vi "SERIAL_DecodePacket.vi"(10 "Data":u8[](array[numeric]), 11 "Packet":string) -> (2 "Data":u8[](array[numeric]), 3 "Packet":string)   [LabVIEW 2015, in "navX Library v1 (deprecated).lvlib"]
uses:
  navX Library v1 (deprecated).lvlib
  COMMON/TypeDefs/Value TypeDefs/navX NAVX_CAPABILITY_FLAGS.ctl
  COMMON/TypeDefs/Value TypeDefs/navX Device Registers.ctl
  TypeDefs/SERIAL_Device_Registers.ctl
  COMMON/Util/DataConvert/LabVIEW-to-navX/EncodeUnsignedHundredths.vi
  COMMON/Util/DataConvert/navX-to-LabVIEW/DecodeSignedHundredths.vi
  COMMON/Util/DataConvert/LabVIEW-to-navX/EncodeSignedHundredths.vi
  COMMON/Util/DataConvert/navX-to-LabVIEW/DecodeUInt16.vi
  COMMON/Util/DataConvert/navX-to-LabVIEW/DecodeInt16.vi
  COMMON/Util/DataConvert/navX-to-LabVIEW/DecodeUInt8.vi
  COMMON/Util/DataConvert/LabVIEW-to-navX/EncodeUInt16.vi
  COMMON/Util/DataConvert/navX-to-LabVIEW/DecodeUnsignedHundredths.vi
  COMMON/Util/DataConvert/navX-to-LabVIEW/DecodeSignedThousandths.vi
  COMMON/Util/DataConvert/LabVIEW-to-navX/EncodeSignedThousandths.vi
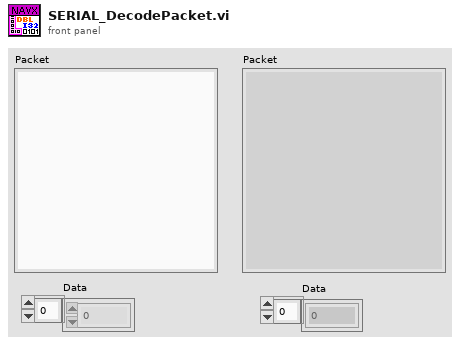
[diagram p1: front panel]
types:
  T1 = typedef "navX Library v1 (deprecated).lvlib/navX Device Registers.ctl" = u8
  T2 = typedef "navX Library v1 (deprecated).lvlib/navX NAVX_CAPABILITY_FLAGS.ctl" = u8
  T3 = typedef "navX Library v1 (deprecated).lvlib/SERIAL_Device_Registers.ctl" = u8
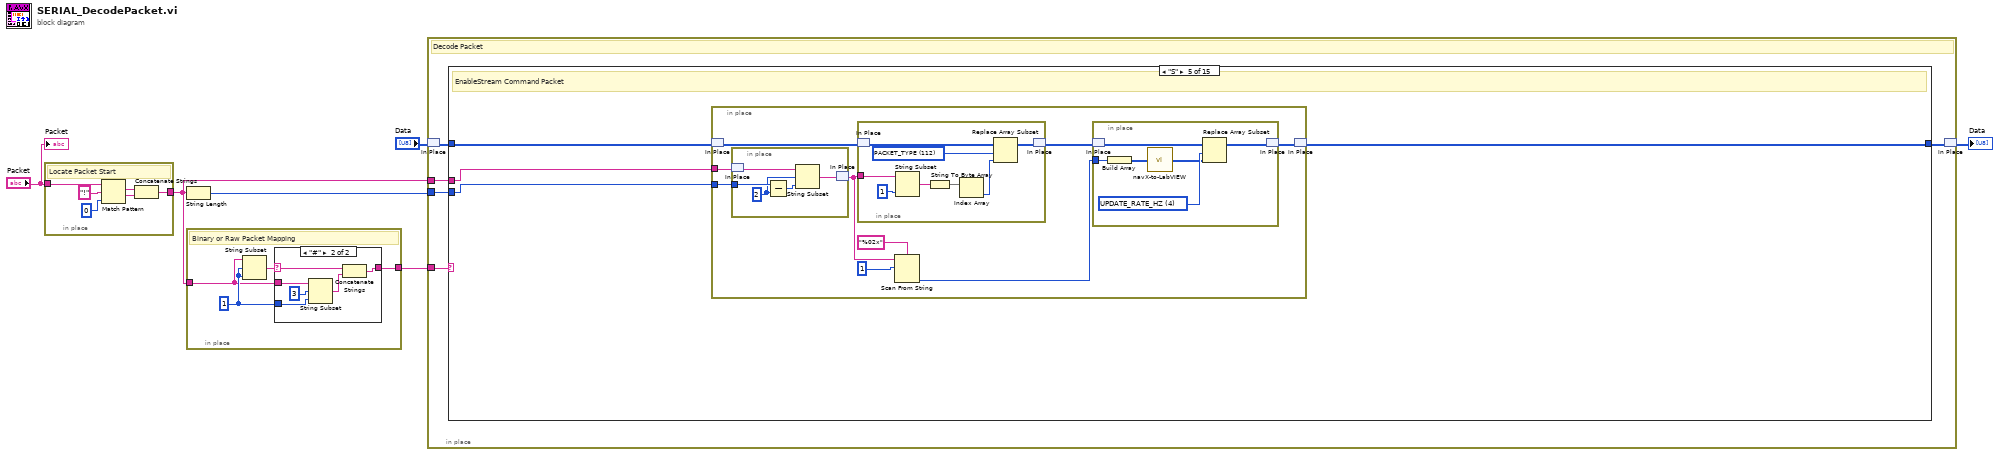
[diagram p0: block diagram]
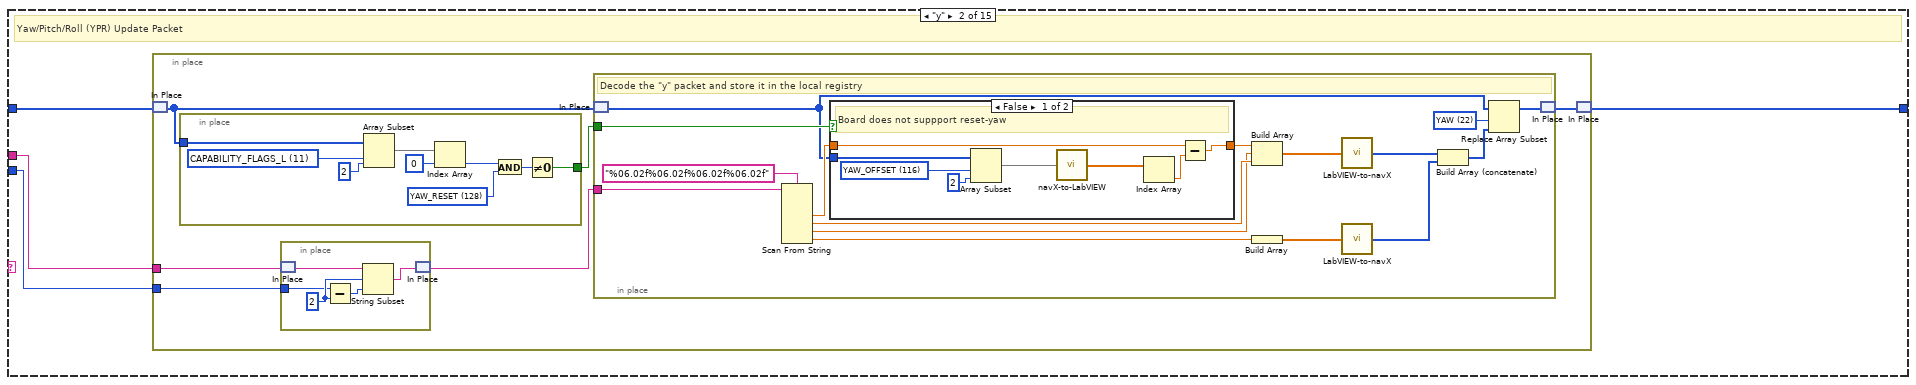
[diagram p3: hidden frame]
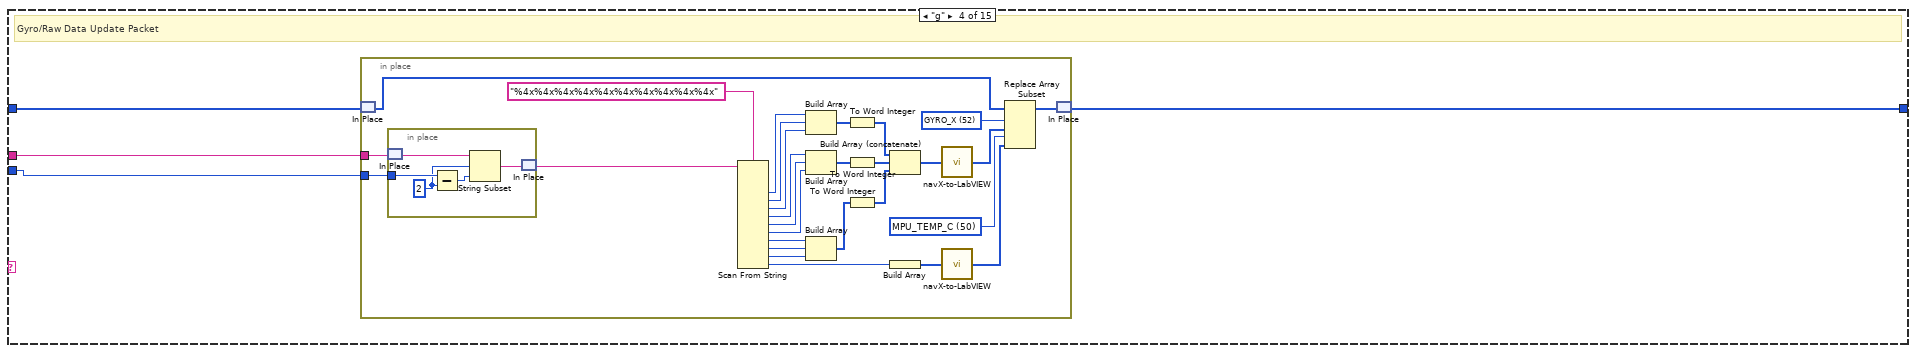
[diagram p6: hidden frame]
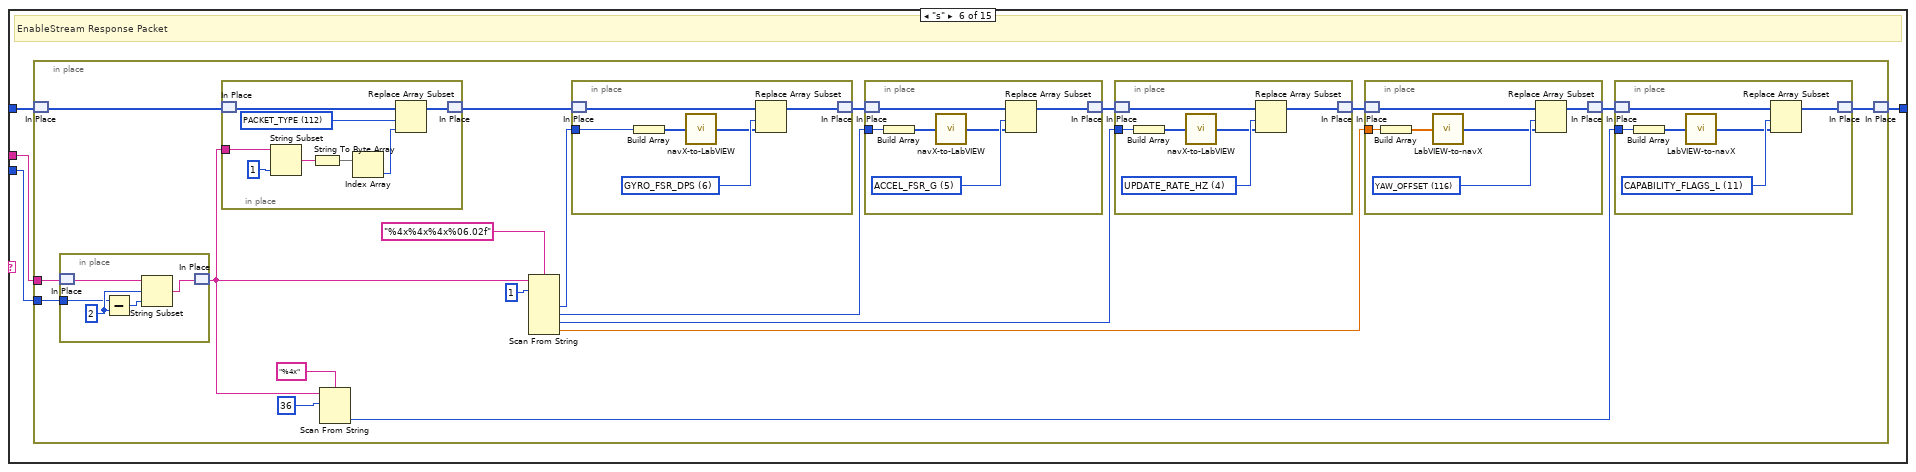
[diagram p7: hidden frame]
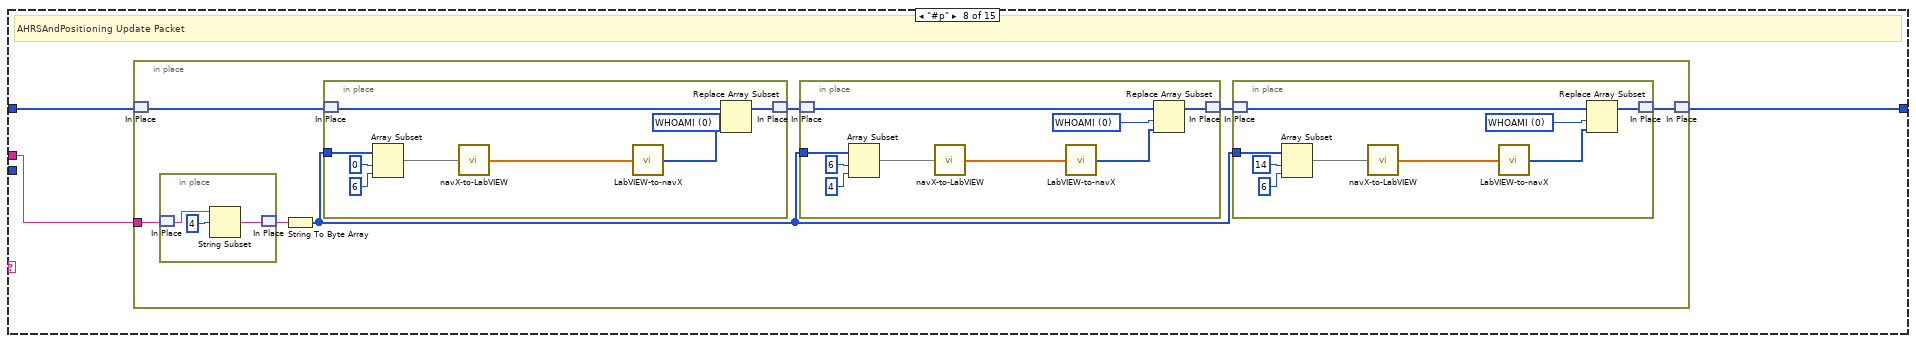
[diagram p9: hidden frame]
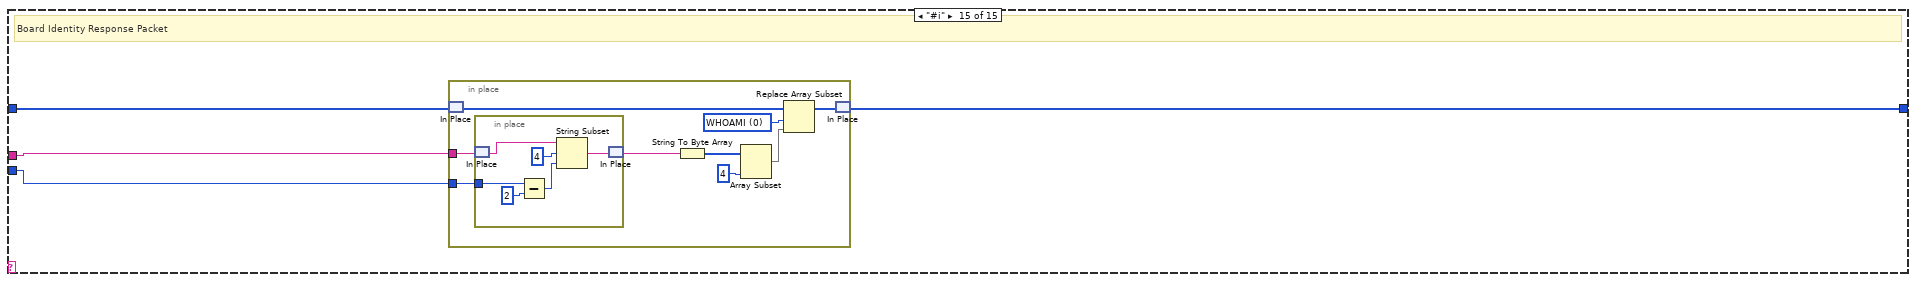
[diagram p16: hidden frame]
diagram:
  n1 = in-place {
    in-place-border: "Packet" -> [w11]
    in-place-border: [w8] -> w4
    # "Locate Packet Start"
    n2 = Match Pattern(string=w11, regular expression="!" ("Packet Start Char"), offset (0)=0 ("offset past match")) -> (match substring=w10:string, after substring=w9:string)  [unwired: 2 out]
    n3 = Concatenate Strings(w10, w9) -> (w8:string)
  }
  n4 = String Length(string=w4) -> (length=w3:i32)
  n5 = in-place {
    in-place-border: w4 -> [w14]
    in-place-border: [w16] -> w6
    w15 = 1 ("length (rest)")
    # "Binary or Raw Packet Mapping"
    n6 = String Subset(string=w14, offset (0)=w15, length (rest)=w15) -> (substring=w13:string)
    n7 = case shown="\"#\"" w13 {
      selector: w13 -> [w17 w18]
      tunnel: [w17 w19] -> w16
      tunnel: w15 -> [_ w22]
      tunnel: w14 -> [_ w21]
      frame Default {
      }
      frame "#" {
        n8 = String Subset(string=w21, offset (0)=3, length (rest)=w22) -> (substring=w20:string)
        n9 = Concatenate Strings(w18, w20) -> (w19:string)
      }
    }
  }
  n10 = in-place {
    in-place-border: w6 -> [w28]
    in-place-border: w4 -> [w27]
    in-place-border: w3 -> [w26]
    # "Decode Packet"
    n11 = in-place-match #1("Data") -> (w25:u8[])
    n12 = case shown="\"S\"" w28 {
      tunnel: w25 -> [w29 w31 w79 w81 w120 w150 w215 w217 w256 w257 w258 w259 w260 w261 w263]
      tunnel: [w29 w30 w79 w80 w119 w149 w215 w216 w256 w257 w258 w259 w260 w261 w262] -> w24
      tunnel: w27 -> [_ w32 _ w83 w118 w152 _ w218 _ _ _ _ _ _ w264]
      tunnel: w26 -> [_ w33 _ w82 w117 w151 _ _ _ _ _ _ _ _ w265]
      frame Default {
        # "Unknown Packet"
      }
      frame "y" {
        # "Yaw/Pitch/Roll (YPR) Update Packet"
        n13 = in-place {
          in-place-border: w33 -> [w38]
          in-place-border: w32 -> [w37]
          n14 = in-place-match #2(w31) -> (w35:u8[])
          n15 = in-place {
            in-place-border: w35 -> [w77]
            in-place-border: [w71] -> w39
            w70 = T1 11 items=["WHOAMI"=0, "HW_REV"=1, "FW_VER_MAJOR"=2, "FW_VER_MINOR"=3, "UPDATE_RATE_HZ"=4, "ACCEL_FSR_G"=5, "GYRO_FSR_DPS"=6, "OP_STATUS"=8, "CAL_STATUS"=9, "SELFTEST_STATUS"=10, "CAPABILITY_FLAGS_L"=11, "CAPABILITY_FLAGS_H"=12, "SENSOR_STATUS"=16, "TIMESTAMP"=18, "YAW"=22, "ROLL"=24, "PITCH"=26, "HEADING"=28, "FUSED_HEADING"=30, "ALTITUDE_I"=32, "ALTITUDE_D"=34, "LINERA_ACC_X"=36, "LINERA_ACC_Y"=38, "LINERA_ACC_Z"=40, "QUAT_W"=42, "QUAT_X"=44, "QUAT_Y"=46, "QUAT_Z"=48, "MPU_TEMP_C"=50, "GYRO_X"=52, "GYRO_Y"=54, "GYRO_Z"=56, "ACC_X"=58, "ACC_Y"=60, "ACC_Z"=62, "MAG_X"=64, "MAG_Y"=66, "MAG_Z"=68, "PRESSURE_I"=70, "PRESSURE_D"=72, "PRESSURE_TEMP"=74, "YAW_OFFSET"=76, "QUAT_OFFSET_W"=78, "QUAT_OFFSET_X"=80, "QUAT_OFFSET_Y"=82, "QUAT_OFFSET_Z"=84, "INTEGRATION_CONTROL"=86, "VELOCITY_X"=88, "VELOCITY_Y"=92, "VELOCITY_Z"=96, "DISPLACMENT_X"=100, "DISPLACMENT_Y"=104, "DISPLACEMENT_Z"=108] ("Device Register")
            w73 = T2 128 items=["OMNIMOUNT"=4, "VEL_AND_DISP "=64, "YAW_RESET"=128, "OMNIMOUNT_CONFIG_MASK"=56] ("NAVX_CAPABILITY_FLAG")
            n16 = Array Subset(array=w77, index=w70, length=2) -> (w75:u8[])
            n17 = Index Array(array=w75, index=u8 0 ("Read Size")) -> (element=w72:u8)
            n18 = And(x=w72, y=w73) -> (x .and. y?=w74:T2)
            n19 = Not Equal To 0?(x=w74) -> (x != 0?=w71:bool)
          }
          n20 = in-place {
            in-place-border: w38 -> [w67]
            w68 = 2 ("offset (0)")
            n21 = in-place-match #3(w37) -> (w65:string)
            n22 = Subtract(x=w67, y=w68) -> (x-y=w69:i32)
            n23 = String Subset(string=w65, offset (0)=w68, length (rest)=w69) -> (substring=w66:string)
            n24 = in-place-match #3(w66) -> (w36:string)
          }
          n25 = in-place {
            in-place-border: w39 -> [w53]
            in-place-border: w36 -> [w43]
            w44 = T1 22 items=["WHOAMI"=0, "HW_REV"=1, "FW_VER_MAJOR"=2, "FW_VER_MINOR"=3, "UPDATE_RATE_HZ"=4, "ACCEL_FSR_G"=5, "GYRO_FSR_DPS"=6, "OP_STATUS"=8, "CAL_STATUS"=9, "SELFTEST_STATUS"=10, "CAPABILITY_FLAGS_L"=11, "CAPABILITY_FLAGS_H"=12, "SENSOR_STATUS"=16, "TIMESTAMP"=18, "YAW"=22, "ROLL"=24, "PITCH"=26, "HEADING"=28, "FUSED_HEADING"=30, "ALTITUDE_I"=32, "ALTITUDE_D"=34, "LINERA_ACC_X"=36, "LINERA_ACC_Y"=38, "LINERA_ACC_Z"=40, "QUAT_W"=42, "QUAT_X"=44, "QUAT_Y"=46, "QUAT_Z"=48, "MPU_TEMP_C"=50, "GYRO_X"=52, "GYRO_Y"=54, "GYRO_Z"=56, "ACC_X"=58, "ACC_Y"=60, "ACC_Z"=62, "MAG_X"=64, "MAG_Y"=66, "MAG_Z"=68, "PRESSURE_I"=70, "PRESSURE_D"=72, "PRESSURE_TEMP"=74, "YAW_OFFSET"=76, "QUAT_OFFSET_W"=78, "QUAT_OFFSET_X"=80, "QUAT_OFFSET_Y"=82, "QUAT_OFFSET_Z"=84, "INTEGRATION_CONTROL"=86, "VELOCITY_X"=88, "VELOCITY_Y"=92, "VELOCITY_Z"=96, "DISPLACMENT_X"=100, "DISPLACMENT_Y"=104, "DISPLACEMENT_Z"=108] ("Device Register")
            # "Decode the \"y\" packet and store it in the local registry"
            n26 = in-place-match #4(w35) -> (w42:u8[])
            n27 = Scan From String(format string="%06.02f%06.02f%06.02f%06.02f", input string=w43) -> (output 1=w54:dbl, output 2=w46:dbl, output 3=w45:dbl, output 4=w48:dbl)  [unwired: 6 in, 3 out]
            n28 = case shown="False" w53 {
              tunnel: [w62 w64] -> w40
              tunnel: w54 -> [w63 w64]
              tunnel: w42 -> [w58 _]
              frame False {
                w60 = T3 116 items=["PACKET_TYPE"=112, "YAW_OFFSET"=116, "ROLL_OFFSET"=118, "PITCH_OFFSET"=120] ("Serial Device Register")
                # "Board does not suppport reset-yaw"
                n29 = Array Subset(array=w58, index=w60, length=2) -> (w59:u8[])
                n30 = call-poly "navX-to-LabVIEW.vi"("Data In"=w59) -> ("Data Out"=w57:dbl[])
                n31 = Index Array(array=w57) -> (element=w56:dbl)  [unwired: 1 in]
                n32 = Subtract(x=w63, y=w56) -> (x-y=w62:dbl)
              }
              frame True {
                # "Board does  suppport reset-yaw"
              }
            }
            n33 = Build Array(w40, w45, w46) -> (w52:dbl[])
            n34 = Build Array(w48) -> (w47:dbl[])
            n35 = call-poly "LabVIEW-to-navX.vi"("Data In"=w52) -> ("Data Out"=w51:u8[])
            n36 = call-poly "LabVIEW-to-navX.vi"("Data In"=w47) -> ("Data Out"=w50:u8[])
            n37 = Build Array (concatenate)(w51, w50) -> (w49:u8[])
            n38 = Replace Array Subset(array=w42, new element=w49, index=w44) -> (w41:u8[])
            n39 = in-place-match #4(w41) -> (w34:u8[])
          }
          n40 = in-place-match #2(w34) -> (w30:u8[])
        }
      }
      frame "q" {
        # "Quaternion Update Packet"
      }
      frame "g" {
        # "Gyro/Raw Data Update Packet"
        n41 = in-place {
          in-place-border: w83 -> [w85]
          in-place-border: w82 -> [w110]
          w88 = T1 50 items=["WHOAMI"=0, "HW_REV"=1, "FW_VER_MAJOR"=2, "FW_VER_MINOR"=3, "UPDATE_RATE_HZ"=4, "ACCEL_FSR_G"=5, "GYRO_FSR_DPS"=6, "OP_STATUS"=8, "CAL_STATUS"=9, "SELFTEST_STATUS"=10, "CAPABILITY_FLAGS_L"=11, "CAPABILITY_FLAGS_H"=12, "SENSOR_STATUS"=16, "TIMESTAMP"=18, "YAW"=22, "PITCH"=24, "ROLL"=26, "HEADING"=28, "FUSED_HEADING"=30, "ALTITUDE_I"=32, "ALTITUDE_D"=34, "LINERA_ACC_X"=36, "LINERA_ACC_Y"=38, "LINERA_ACC_Z"=40, "QUAT_W"=42, "QUAT_X"=44, "QUAT_Y"=46, "QUAT_Z"=48, "MPU_TEMP_C"=50, "GYRO_X"=52, "GYRO_Y"=54, "GYRO_Z"=56, "ACC_X"=58, "ACC_Y"=60, "ACC_Z"=62, "MAG_X"=64, "MAG_Y"=66, "MAG_Z"=68, "PRESSURE_I"=70, "PRESSURE_D"=72, "PRESSURE_TEMP"=74, "YAW_OFFSET"=76, "QUAT_OFFSET_W"=78, "QUAT_OFFSET_X"=80, "QUAT_OFFSET_Y"=82, "QUAT_OFFSET_Z"=84, "INTEGRATION_CONTROL"=86, "VELOCITY_X"=88, "VELOCITY_Y"=92, "VELOCITY_Z"=96, "DISPLACMENT_X"=100, "DISPLACMENT_Y"=104, "DISPLACEMENT_Z"=108] ("Device Register")
          w111 = T1 52 items=["WHOAMI"=0, "HW_REV"=1, "FW_VER_MAJOR"=2, "FW_VER_MINOR"=3, "UPDATE_RATE_HZ"=4, "ACCEL_FSR_G"=5, "GYRO_FSR_DPS"=6, "OP_STATUS"=8, "CAL_STATUS"=9, "SELFTEST_STATUS"=10, "CAPABILITY_FLAGS_L"=11, "CAPABILITY_FLAGS_H"=12, "SENSOR_STATUS"=16, "TIMESTAMP"=18, "YAW"=22, "PITCH"=24, "ROLL"=26, "HEADING"=28, "FUSED_HEADING"=30, "ALTITUDE_I"=32, "ALTITUDE_D"=34, "LINERA_ACC_X"=36, "LINERA_ACC_Y"=38, "LINERA_ACC_Z"=40, "QUAT_W"=42, "QUAT_X"=44, "QUAT_Y"=46, "QUAT_Z"=48, "MPU_TEMP_C"=50, "GYRO_X"=52, "GYRO_Y"=54, "GYRO_Z"=56, "ACC_X"=58, "ACC_Y"=60, "ACC_Z"=62, "MAG_X"=64, "MAG_Y"=66, "MAG_Z"=68, "PRESSURE_I"=70, "PRESSURE_D"=72, "PRESSURE_TEMP"=74, "YAW_OFFSET"=76, "QUAT_OFFSET_W"=78, "QUAT_OFFSET_X"=80, "QUAT_OFFSET_Y"=82, "QUAT_OFFSET_Z"=84, "INTEGRATION_CONTROL"=86, "VELOCITY_X"=88, "VELOCITY_Y"=92, "VELOCITY_Z"=96, "DISPLACMENT_X"=100, "DISPLACMENT_Y"=104, "DISPLACEMENT_Z"=108] ("Device Register")
          n42 = in-place-match #5(w81) -> (w93:u8[])
          n43 = in-place {
            in-place-border: w110 -> [w116]
            w114 = 2 ("offset (0)")
            n44 = in-place-match #6(w85) -> (w113:string)
            n45 = Subtract(x=w116, y=w114) -> (x-y=w115:i32)
            n46 = String Subset(string=w113, offset (0)=w114, length (rest)=w115) -> (substring=w112:string)
            n47 = in-place-match #6(w112) -> (w84:string)
          }
          n48 = Scan From String(format string="%4x%4x%4x%4x%4x%4x%4x%4x%4x%4x", input string=w84) -> (output 1=w108:u32, output 2=w107:u32, output 3=w106:u32, output 4=w105:u32, output 5=w104:u32, output 6=w103:u32, output 7=w102:u32, output 8=w101:u32, output 9=w100:u32, output 10=w91:u32)  [unwired: 12 in, 3 out]
          n49 = Build Array(w108, w107, w106) -> (w97:u32[])
          n50 = Build Array(w105, w104, w103) -> (w99:u32[])
          n51 = Build Array(w102, w101, w100) -> (w98:u32[])
          n52 = To Word Integer(number=w97) -> (16bit integer=w96:i16[])
          n53 = To Word Integer(number=w99) -> (16bit integer=w95:i16[])
          n54 = To Word Integer(number=w98) -> (16bit integer=w92:i16[])
          n55 = Build Array (concatenate)(w96, w95, w92) -> (w87:i16[])
          n56 = Build Array(w91) -> (w90:u32[])
          n57 = call-poly "navX-to-LabVIEW.vi"("Data In"=w87) -> ("Data Out"=w86:i16[])
          n58 = call-poly "navX-to-LabVIEW.vi"("Data In"=w90) -> ("Data Out"=w89:u16[])
          n59 = Replace Array Subset(array=w93, new element #1=w86, index #1=w111, new element #2=w89, index #2=w88) -> (w94:u8[])
          n60 = in-place-match #5(w94) -> (w80:u8[])
        }
      }
      frame "S" {
        # "EnableStream Command Packet"
        n61 = in-place {
          in-place-border: w118 -> [w128]
          in-place-border: w117 -> [w127]
          n62 = in-place-match #7(w120) -> (w129:u8[])
          n63 = in-place {
            in-place-border: w127 -> [w140]
            w138 = 2 ("offset (0)")
            n64 = in-place-match #8(w128) -> (w137:string)
            n65 = Subtract(x=w140, y=w138) -> (x-y=w139:i32)
            n66 = String Subset(string=w137, offset (0)=w138, length (rest)=w139) -> (substring=w136:string)
            n67 = in-place-match #8(w136) -> (w126:string)
          }
          n68 = in-place {
            in-place-border: w126 -> [w148]
            w143 = T3 112 items=["PACKET_TYPE"=112, "YAW_OFFSET"=116, "ROLL_OFFSET"=118, "PITCH_OFFSET"=120] ("Serial Device Register")
            n69 = in-place-match #9(w129) -> (w144:u8[])
            n70 = String Subset(string=w148, length (rest)=1 ("length (rest)")) -> (substring=w146:string)  [unwired: 1 in]
            n71 = String To Byte Array(string=w146) -> (unsigned byte array=w145:u8[])
            n72 = Index Array(array=w145) -> (element=w142:u8)  [unwired: 1 in]
            n73 = Replace Array Subset(array=w144, new element=w142, index=w143) -> (w141:u8[])
            n74 = in-place-match #9(w141) -> (w121:u8[])
          }
          n75 = Scan From String(format string="%02x", input string=w126, initial scan location=u32 1) -> (output 1=w123:u32)  [unwired: 2 in, 3 out]
          n76 = in-place {
            in-place-border: w123 -> [w135]
            w133 = T1 4 items=["WHOAMI"=0, "HW_REV"=1, "FW_VER_MAJOR"=2, "FW_VER_MINOR"=3, "UPDATE_RATE_HZ"=4, "ACCEL_FSR_G"=5, "GYRO_FSR_DPS"=6, "OP_STATUS"=8, "CAL_STATUS"=9, "SELFTEST_STATUS"=10, "CAPABILITY_FLAGS_L"=11, "CAPABILITY_FLAGS_H"=12, "SENSOR_STATUS"=16, "TIMESTAMP"=18, "YAW"=22, "PITCH"=24, "ROLL"=26, "HEADING"=28, "FUSED_HEADING"=30, "ALTITUDE_I"=32, "ALTITUDE_D"=34, "LINERA_ACC_X"=36, "LINERA_ACC_Y"=38, "LINERA_ACC_Z"=40, "QUAT_W"=42, "QUAT_X"=44, "QUAT_Y"=46, "QUAT_Z"=48, "MPU_TEMP_C"=50, "GYRO_X"=52, "GYRO_Y"=54, "GYRO_Z"=56, "ACC_X"=58, "ACC_Y"=60, "ACC_Z"=62, "MAG_X"=64, "MAG_Y"=66, "MAG_Z"=68, "PRESSURE_I"=70, "PRESSURE_D"=72, "PRESSURE_TEMP"=74, "YAW_OFFSET"=76, "QUAT_OFFSET_W"=78, "QUAT_OFFSET_X"=80, "QUAT_OFFSET_Y"=82, "QUAT_OFFSET_Z"=84, "INTEGRATION_CONTROL"=86, "VELOCITY_X"=88, "VELOCITY_Y"=92, "VELOCITY_Z"=96, "DISPLACMENT_X"=100, "DISPLACMENT_Y"=104, "DISPLACEMENT_Z"=108] ("Device Register")
            n77 = in-place-match #10(w121) -> (w131:u8[])
            n78 = Build Array(w135) -> (w134:u32[])
            n79 = call-poly "navX-to-LabVIEW.vi"("Data In"=w134) -> ("Data Out"=w132:u8[])
            n80 = Replace Array Subset(array=w131, new element=w132, index=w133) -> (w130:u8[])
            n81 = in-place-match #10(w130) -> (w122:u8[])
          }
          n82 = in-place-match #7(w122) -> (w119:u8[])
        }
      }
      frame "s" {
        # "EnableStream Response Packet"
        n83 = in-place {
          in-place-border: w152 -> [w166]
          in-place-border: w151 -> [w170]
          n84 = in-place-match #11(w150) -> (w165:u8[])
          n85 = in-place {
            in-place-border: w170 -> [w212]
            w213 = 2 ("offset (0)")
            n86 = in-place-match #12(w166) -> (w211:string)
            n87 = Subtract(x=w212, y=w213) -> (x-y=w214:i32)
            n88 = String Subset(string=w211, offset (0)=w213, length (rest)=w214) -> (substring=w210:string)
            n89 = in-place-match #12(w210) -> (w164:string)
          }
          n90 = in-place {
            in-place-border: w164 -> [w209]
            w204 = T3 112 items=["PACKET_TYPE"=112, "YAW_OFFSET"=116, "ROLL_OFFSET"=118, "PITCH_OFFSET"=120] ("Serial Device Register")
            n91 = in-place-match #13(w165) -> (w205:u8[])
            n92 = String Subset(string=w209, length (rest)=1 ("length (rest)")) -> (substring=w207:string)  [unwired: 1 in]
            n93 = String To Byte Array(string=w207) -> (unsigned byte array=w206:u8[])
            n94 = Index Array(array=w206) -> (element=w203:u8)  [unwired: 1 in]
            n95 = Replace Array Subset(array=w205, new element=w203, index=w204) -> (w202:u8[])
            n96 = in-place-match #13(w202) -> (w163:u8[])
          }
          n97 = Scan From String(format string="%4x", input string=w164, initial scan location=u32 36) -> (output 1=w154:u32)  [unwired: 2 in, 3 out]
          n98 = Scan From String(format string="%4x%4x%4x%06.02f", input string=w164, initial scan location=u32 1) -> (output 1=w161:u32, output 2=w160:u32, output 3=w158:u32, output 4=w156:dbl)  [unwired: 5 in, 3 out]
          n99 = in-place {
            in-place-border: w161 -> [w201]
            w199 = T1 6 items=["WHOAMI"=0, "HW_REV"=1, "FW_VER_MAJOR"=2, "FW_VER_MINOR"=3, "UPDATE_RATE_HZ"=4, "ACCEL_FSR_G"=5, "GYRO_FSR_DPS"=6, "OP_STATUS"=8, "CAL_STATUS"=9, "SELFTEST_STATUS"=10, "CAPABILITY_FLAGS_L"=11, "CAPABILITY_FLAGS_H"=12, "SENSOR_STATUS"=16, "TIMESTAMP"=18, "YAW"=22, "PITCH"=24, "ROLL"=26, "HEADING"=28, "FUSED_HEADING"=30, "ALTITUDE_I"=32, "ALTITUDE_D"=34, "LINERA_ACC_X"=36, "LINERA_ACC_Y"=38, "LINERA_ACC_Z"=40, "QUAT_W"=42, "QUAT_X"=44, "QUAT_Y"=46, "QUAT_Z"=48, "MPU_TEMP_C"=50, "GYRO_X"=52, "GYRO_Y"=54, "GYRO_Z"=56, "ACC_X"=58, "ACC_Y"=60, "ACC_Z"=62, "MAG_X"=64, "MAG_Y"=66, "MAG_Z"=68, "PRESSURE_I"=70, "PRESSURE_D"=72, "PRESSURE_TEMP"=74, "YAW_OFFSET"=76, "QUAT_OFFSET_W"=78, "QUAT_OFFSET_X"=80, "QUAT_OFFSET_Y"=82, "QUAT_OFFSET_Z"=84, "INTEGRATION_CONTROL"=86, "VELOCITY_X"=88, "VELOCITY_Y"=92, "VELOCITY_Z"=96, "DISPLACMENT_X"=100, "DISPLACMENT_Y"=104, "DISPLACEMENT_Z"=108] ("Device Register")
            n100 = in-place-match #14(w163) -> (w197:u8[])
            n101 = Build Array(w201) -> (w200:u32[])
            n102 = call-poly "navX-to-LabVIEW.vi"("Data In"=w200) -> ("Data Out"=w198:u16[])
            n103 = Replace Array Subset(array=w197, new element=w198, index=w199) -> (w196:u8[])
            n104 = in-place-match #14(w196) -> (w162:u8[])
          }
          n105 = in-place {
            in-place-border: w160 -> [w195]
            w193 = T1 5 items=["WHOAMI"=0, "HW_REV"=1, "FW_VER_MAJOR"=2, "FW_VER_MINOR"=3, "UPDATE_RATE_HZ"=4, "ACCEL_FSR_G"=5, "GYRO_FSR_DPS"=6, "OP_STATUS"=8, "CAL_STATUS"=9, "SELFTEST_STATUS"=10, "CAPABILITY_FLAGS_L"=11, "CAPABILITY_FLAGS_H"=12, "SENSOR_STATUS"=16, "TIMESTAMP"=18, "YAW"=22, "PITCH"=24, "ROLL"=26, "HEADING"=28, "FUSED_HEADING"=30, "ALTITUDE_I"=32, "ALTITUDE_D"=34, "LINERA_ACC_X"=36, "LINERA_ACC_Y"=38, "LINERA_ACC_Z"=40, "QUAT_W"=42, "QUAT_X"=44, "QUAT_Y"=46, "QUAT_Z"=48, "MPU_TEMP_C"=50, "GYRO_X"=52, "GYRO_Y"=54, "GYRO_Z"=56, "ACC_X"=58, "ACC_Y"=60, "ACC_Z"=62, "MAG_X"=64, "MAG_Y"=66, "MAG_Z"=68, "PRESSURE_I"=70, "PRESSURE_D"=72, "PRESSURE_TEMP"=74, "YAW_OFFSET"=76, "QUAT_OFFSET_W"=78, "QUAT_OFFSET_X"=80, "QUAT_OFFSET_Y"=82, "QUAT_OFFSET_Z"=84, "INTEGRATION_CONTROL"=86, "VELOCITY_X"=88, "VELOCITY_Y"=92, "VELOCITY_Z"=96, "DISPLACMENT_X"=100, "DISPLACMENT_Y"=104, "DISPLACEMENT_Z"=108] ("Device Register")
            n106 = in-place-match #15(w162) -> (w191:u8[])
            n107 = Build Array(w195) -> (w194:u32[])
            n108 = call-poly "navX-to-LabVIEW.vi"("Data In"=w194) -> ("Data Out"=w192:u16[])
            n109 = Replace Array Subset(array=w191, new element=w192, index=w193) -> (w190:u8[])
            n110 = in-place-match #15(w190) -> (w159:u8[])
          }
          n111 = in-place {
            in-place-border: w158 -> [w189]
            w187 = T1 4 items=["WHOAMI"=0, "HW_REV"=1, "FW_VER_MAJOR"=2, "FW_VER_MINOR"=3, "UPDATE_RATE_HZ"=4, "ACCEL_FSR_G"=5, "GYRO_FSR_DPS"=6, "OP_STATUS"=8, "CAL_STATUS"=9, "SELFTEST_STATUS"=10, "CAPABILITY_FLAGS_L"=11, "CAPABILITY_FLAGS_H"=12, "SENSOR_STATUS"=16, "TIMESTAMP"=18, "YAW"=22, "PITCH"=24, "ROLL"=26, "HEADING"=28, "FUSED_HEADING"=30, "ALTITUDE_I"=32, "ALTITUDE_D"=34, "LINERA_ACC_X"=36, "LINERA_ACC_Y"=38, "LINERA_ACC_Z"=40, "QUAT_W"=42, "QUAT_X"=44, "QUAT_Y"=46, "QUAT_Z"=48, "MPU_TEMP_C"=50, "GYRO_X"=52, "GYRO_Y"=54, "GYRO_Z"=56, "ACC_X"=58, "ACC_Y"=60, "ACC_Z"=62, "MAG_X"=64, "MAG_Y"=66, "MAG_Z"=68, "PRESSURE_I"=70, "PRESSURE_D"=72, "PRESSURE_TEMP"=74, "YAW_OFFSET"=76, "QUAT_OFFSET_W"=78, "QUAT_OFFSET_X"=80, "QUAT_OFFSET_Y"=82, "QUAT_OFFSET_Z"=84, "INTEGRATION_CONTROL"=86, "VELOCITY_X"=88, "VELOCITY_Y"=92, "VELOCITY_Z"=96, "DISPLACMENT_X"=100, "DISPLACMENT_Y"=104, "DISPLACEMENT_Z"=108] ("Device Register")
            n112 = in-place-match #16(w159) -> (w185:u8[])
            n113 = Build Array(w189) -> (w188:u32[])
            n114 = call-poly "navX-to-LabVIEW.vi"("Data In"=w188) -> ("Data Out"=w186:u8[])
            n115 = Replace Array Subset(array=w185, new element=w186, index=w187) -> (w184:u8[])
            n116 = in-place-match #16(w184) -> (w157:u8[])
          }
          n117 = in-place {
            in-place-border: w156 -> [w183]
            w181 = T3 116 items=["PACKET_TYPE"=112, "YAW_OFFSET"=116, "ROLL_OFFSET"=118, "PITCH_OFFSET"=120] ("Serial Device Register")
            n118 = in-place-match #17(w157) -> (w179:u8[])
            n119 = Build Array(w183) -> (w182:dbl[])
            n120 = call-poly "LabVIEW-to-navX.vi"("Data In"=w182) -> ("Data Out"=w180:u8[])
            n121 = Replace Array Subset(array=w179, new element=w180, index=w181) -> (w178:u8[])
            n122 = in-place-match #17(w178) -> (w155:u8[])
          }
          n123 = in-place {
            in-place-border: w154 -> [w177]
            w175 = T1 11 items=["WHOAMI"=0, "HW_REV"=1, "FW_VER_MAJOR"=2, "FW_VER_MINOR"=3, "UPDATE_RATE_HZ"=4, "ACCEL_FSR_G"=5, "GYRO_FSR_DPS"=6, "OP_STATUS"=8, "CAL_STATUS"=9, "SELFTEST_STATUS"=10, "CAPABILITY_FLAGS_L"=11, "CAPABILITY_FLAGS_H"=12, "SENSOR_STATUS"=16, "TIMESTAMP"=18, "YAW"=22, "PITCH"=24, "ROLL"=26, "HEADING"=28, "FUSED_HEADING"=30, "ALTITUDE_I"=32, "ALTITUDE_D"=34, "LINERA_ACC_X"=36, "LINERA_ACC_Y"=38, "LINERA_ACC_Z"=40, "QUAT_W"=42, "QUAT_X"=44, "QUAT_Y"=46, "QUAT_Z"=48, "MPU_TEMP_C"=50, "GYRO_X"=52, "GYRO_Y"=54, "GYRO_Z"=56, "ACC_X"=58, "ACC_Y"=60, "ACC_Z"=62, "MAG_X"=64, "MAG_Y"=66, "MAG_Z"=68, "PRESSURE_I"=70, "PRESSURE_D"=72, "PRESSURE_TEMP"=74, "YAW_OFFSET"=76, "QUAT_OFFSET_W"=78, "QUAT_OFFSET_X"=80, "QUAT_OFFSET_Y"=82, "QUAT_OFFSET_Z"=84, "INTEGRATION_CONTROL"=86, "VELOCITY_X"=88, "VELOCITY_Y"=92, "VELOCITY_Z"=96, "DISPLACMENT_X"=100, "DISPLACMENT_Y"=104, "DISPLACEMENT_Z"=108] ("Device Register")
            n124 = in-place-match #18(w155) -> (w173:u8[])
            n125 = Build Array(w177) -> (w176:u32[])
            n126 = call-poly "LabVIEW-to-navX.vi"("Data In"=w176) -> ("Data Out"=w174:u8[])
            n127 = Replace Array Subset(array=w173, new element=w174, index=w175) -> (w172:u8[])
            n128 = in-place-match #18(w172) -> (w153:u8[])
          }
          n129 = in-place-match #11(w153) -> (w149:u8[])
        }
      }
      frame "#a" {
        # "AHRS Update Packet"
      }
      frame "#p" {
        # "AHRSAndPositioning Update Packet"
        n130 = in-place {
          in-place-border: w218 -> [w222]
          n131 = in-place-match #19(w217) -> (w220:u8[])
          n132 = in-place {
            n133 = in-place-match #20(w222) -> (w228:string)
            n134 = String Subset(string=w228, offset (0)=4) -> (substring=w226:string)  [unwired: 1 in]
            n135 = in-place-match #20(w226) -> (w221:string)
          }
          n136 = String To Byte Array(string=w221) -> (unsigned byte array=w223:u8[])
          n137 = in-place {
            in-place-border: w223 -> [w252]
            w247 = T1 0 items=["WHOAMI"=0, "HW_REV"=1, "FW_VER_MAJOR"=2, "FW_VER_MINOR"=3, "UPDATE_RATE_HZ"=4, "ACCEL_FSR_G"=5, "GYRO_FSR_DPS"=6, "OP_STATUS"=8, "CAL_STATUS"=9, "SELFTEST_STATUS"=10, "CAPABILITY_FLAGS_L"=11, "CAPABILITY_FLAGS_H"=12, "SENSOR_STATUS"=16, "TIMESTAMP"=18, "YAW"=22, "PITCH"=24, "ROLL"=26, "HEADING"=28, "FUSED_HEADING"=30, "ALTITUDE_I"=32, "ALTITUDE_D"=34, "LINERA_ACC_X"=36, "LINERA_ACC_Y"=38, "LINERA_ACC_Z"=40, "QUAT_W"=42, "QUAT_X"=44, "QUAT_Y"=46, "QUAT_Z"=48, "MPU_TEMP_C"=50, "GYRO_X"=52, "GYRO_Y"=54, "GYRO_Z"=56, "ACC_X"=58, "ACC_Y"=60, "ACC_Z"=62, "MAG_X"=64, "MAG_Y"=66, "MAG_Z"=68, "PRESSURE_I"=70, "PRESSURE_D"=72, "PRESSURE_TEMP"=74, "YAW_OFFSET"=76, "QUAT_OFFSET_W"=78, "QUAT_OFFSET_X"=80, "QUAT_OFFSET_Y"=82, "QUAT_OFFSET_Z"=84, "INTEGRATION_CONTROL"=86, "VELOCITY_X"=88, "VELOCITY_Y"=92, "VELOCITY_Z"=96, "DISPLACMENT_X"=100, "DISPLACMENT_Y"=104, "DISPLACEMENT_Z"=108] ("Device Register")
            n138 = in-place-match #21(w220) -> (w250:u8[])
            n139 = Array Subset(array=w252, index=0, length=6) -> (w255:u8[])
            n140 = call-poly "navX-to-LabVIEW.vi"("Data In"=w255) -> ("Data Out"=w251:dbl[])
            n141 = call-poly "LabVIEW-to-navX.vi"("Data In"=w251) -> ("Data Out"=w249:u8[])
            n142 = Replace Array Subset(array=w250, new element=w249, index=w247) -> (w248:u8[])
            n143 = in-place-match #21(w248) -> (w225:u8[])
          }
          n144 = in-place {
            in-place-border: w223 -> [w243]
            w238 = T1 0 items=["WHOAMI"=0, "HW_REV"=1, "FW_VER_MAJOR"=2, "FW_VER_MINOR"=3, "UPDATE_RATE_HZ"=4, "ACCEL_FSR_G"=5, "GYRO_FSR_DPS"=6, "OP_STATUS"=8, "CAL_STATUS"=9, "SELFTEST_STATUS"=10, "CAPABILITY_FLAGS_L"=11, "CAPABILITY_FLAGS_H"=12, "SENSOR_STATUS"=16, "TIMESTAMP"=18, "YAW"=22, "PITCH"=24, "ROLL"=26, "HEADING"=28, "FUSED_HEADING"=30, "ALTITUDE_I"=32, "ALTITUDE_D"=34, "LINERA_ACC_X"=36, "LINERA_ACC_Y"=38, "LINERA_ACC_Z"=40, "QUAT_W"=42, "QUAT_X"=44, "QUAT_Y"=46, "QUAT_Z"=48, "MPU_TEMP_C"=50, "GYRO_X"=52, "GYRO_Y"=54, "GYRO_Z"=56, "ACC_X"=58, "ACC_Y"=60, "ACC_Z"=62, "MAG_X"=64, "MAG_Y"=66, "MAG_Z"=68, "PRESSURE_I"=70, "PRESSURE_D"=72, "PRESSURE_TEMP"=74, "YAW_OFFSET"=76, "QUAT_OFFSET_W"=78, "QUAT_OFFSET_X"=80, "QUAT_OFFSET_Y"=82, "QUAT_OFFSET_Z"=84, "INTEGRATION_CONTROL"=86, "VELOCITY_X"=88, "VELOCITY_Y"=92, "VELOCITY_Z"=96, "DISPLACMENT_X"=100, "DISPLACMENT_Y"=104, "DISPLACEMENT_Z"=108] ("Device Register")
            n145 = in-place-match #22(w225) -> (w241:u8[])
            n146 = Array Subset(array=w243, index=6, length=4) -> (w246:u8[])
            n147 = call-poly "navX-to-LabVIEW.vi"("Data In"=w246) -> ("Data Out"=w242:dbl[])
            n148 = call-poly "LabVIEW-to-navX.vi"("Data In"=w242) -> ("Data Out"=w240:u8[])
            n149 = Replace Array Subset(array=w241, new element=w240, index=w238) -> (w239:u8[])
            n150 = in-place-match #22(w239) -> (w224:u8[])
          }
          n151 = in-place {
            in-place-border: w223 -> [w234]
            w229 = T1 0 items=["WHOAMI"=0, "HW_REV"=1, "FW_VER_MAJOR"=2, "FW_VER_MINOR"=3, "UPDATE_RATE_HZ"=4, "ACCEL_FSR_G"=5, "GYRO_FSR_DPS"=6, "OP_STATUS"=8, "CAL_STATUS"=9, "SELFTEST_STATUS"=10, "CAPABILITY_FLAGS_L"=11, "CAPABILITY_FLAGS_H"=12, "SENSOR_STATUS"=16, "TIMESTAMP"=18, "YAW"=22, "PITCH"=24, "ROLL"=26, "HEADING"=28, "FUSED_HEADING"=30, "ALTITUDE_I"=32, "ALTITUDE_D"=34, "LINERA_ACC_X"=36, "LINERA_ACC_Y"=38, "LINERA_ACC_Z"=40, "QUAT_W"=42, "QUAT_X"=44, "QUAT_Y"=46, "QUAT_Z"=48, "MPU_TEMP_C"=50, "GYRO_X"=52, "GYRO_Y"=54, "GYRO_Z"=56, "ACC_X"=58, "ACC_Y"=60, "ACC_Z"=62, "MAG_X"=64, "MAG_Y"=66, "MAG_Z"=68, "PRESSURE_I"=70, "PRESSURE_D"=72, "PRESSURE_TEMP"=74, "YAW_OFFSET"=76, "QUAT_OFFSET_W"=78, "QUAT_OFFSET_X"=80, "QUAT_OFFSET_Y"=82, "QUAT_OFFSET_Z"=84, "INTEGRATION_CONTROL"=86, "VELOCITY_X"=88, "VELOCITY_Y"=92, "VELOCITY_Z"=96, "DISPLACMENT_X"=100, "DISPLACMENT_Y"=104, "DISPLACEMENT_Z"=108] ("Device Register")
            n152 = in-place-match #23(w224) -> (w232:u8[])
            n153 = Array Subset(array=w234, index=14, length=6) -> (w237:u8[])
            n154 = call-poly "navX-to-LabVIEW.vi"("Data In"=w237) -> ("Data Out"=w233:dbl[])
            n155 = call-poly "LabVIEW-to-navX.vi"("Data In"=w233) -> ("Data Out"=w231:u8[])
            n156 = Replace Array Subset(array=w232, new element=w231, index=w229) -> (w230:u8[])
            n157 = in-place-match #23(w230) -> (w219:u8[])
          }
          n158 = in-place-match #19(w219) -> (w216:u8[])
        }
      }
      frame "#D" {
        # "Data Get Request"
      }
      frame "#v" {
        # "Data Set Response Packet"
      }
      frame "#I" {
        # "Integration Control Command Packet"
      }
      frame "#j" {
        # "Integration Control Response Packet"
      }
      frame "#M" {
        # "Magnetometer Calibration Packet"
      }
      frame "#T" {
        # "Tuning Variable Packet"
      }
      frame "#i" {
        # "Board Identity Response Packet"
        n159 = in-place {
          in-place-border: w265 -> [w274]
          in-place-border: w264 -> [w269]
          w273 = T1 0 items=["WHOAMI"=0, "HW_REV"=1, "FW_VER_MAJOR"=2, "FW_VER_MINOR"=3, "UPDATE_RATE_HZ"=4, "ACCEL_FSR_G"=5, "GYRO_FSR_DPS"=6, "OP_STATUS"=8, "CAL_STATUS"=9, "SELFTEST_STATUS"=10, "CAPABILITY_FLAGS_L"=11, "CAPABILITY_FLAGS_H"=12, "SENSOR_STATUS"=16, "TIMESTAMP"=18, "YAW"=22, "PITCH"=24, "ROLL"=26, "HEADING"=28, "FUSED_HEADING"=30, "ALTITUDE_I"=32, "ALTITUDE_D"=34, "LINERA_ACC_X"=36, "LINERA_ACC_Y"=38, "LINERA_ACC_Z"=40, "QUAT_W"=42, "QUAT_X"=44, "QUAT_Y"=46, "QUAT_Z"=48, "MPU_TEMP_C"=50, "GYRO_X"=52, "GYRO_Y"=54, "GYRO_Z"=56, "ACC_X"=58, "ACC_Y"=60, "ACC_Z"=62, "MAG_X"=64, "MAG_Y"=66, "MAG_Z"=68, "PRESSURE_I"=70, "PRESSURE_D"=72, "PRESSURE_TEMP"=74, "YAW_OFFSET"=76, "QUAT_OFFSET_W"=78, "QUAT_OFFSET_X"=80, "QUAT_OFFSET_Y"=82, "QUAT_OFFSET_Z"=84, "INTEGRATION_CONTROL"=86, "VELOCITY_X"=88, "VELOCITY_Y"=92, "VELOCITY_Z"=96, "DISPLACMENT_X"=100, "DISPLACMENT_Y"=104, "DISPLACEMENT_Z"=108] ("Device Register")
          n160 = in-place-match #24(w263) -> (w267:u8[])
          n161 = in-place {
            in-place-border: w274 -> [w280]
            n162 = in-place-match #25(w269) -> (w276:string)
            n163 = Subtract(x=w280, y=2 ("offset (0)")) -> (x-y=w279:i32)
            n164 = String Subset(string=w276, offset (0)=4, length (rest)=w279) -> (substring=w275:string)
            n165 = in-place-match #25(w275) -> (w268:string)
          }
          n166 = String To Byte Array(string=w268) -> (unsigned byte array=w272:u8[])
          n167 = Array Subset(array=w272, length=4) -> (w271:u8[])  [unwired: 1 in]
          n168 = Replace Array Subset(array=w267, new element=w271, index=w273) -> (w266:u8[])
          n169 = in-place-match #24(w266) -> (w262:u8[])
        }
      }
    }
    n170 = in-place-match #1(w24) -> (→"Data":u8[])
  }
  "Packet" <- "Packet"
